vi "PWM_Write.vi"(8 "error in (no error)":errorcluster, 9 "DC":u8(slide) scale=0.0..255.0, 10 "Pin":u8=4 min=4 max=40, 11 "VISA resource name":refnum<visa-resource-name>) -> (0 "error out":errorcluster, 3 "VISA resource name out":refnum<visa-resource-name>)   [LabVIEW 2025]
panel:
  in  "DC%":u8(slide) scale=0.0..100.0
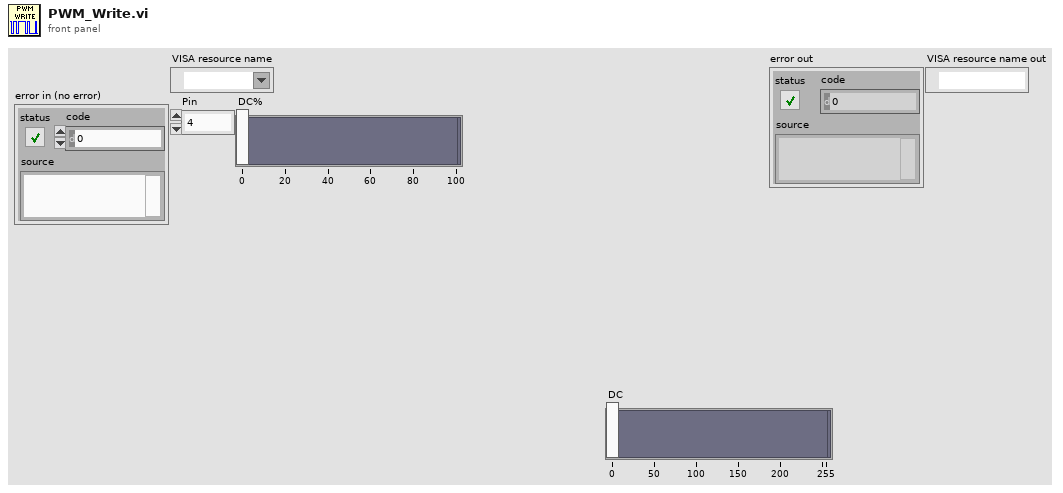
[diagram p1: front panel]
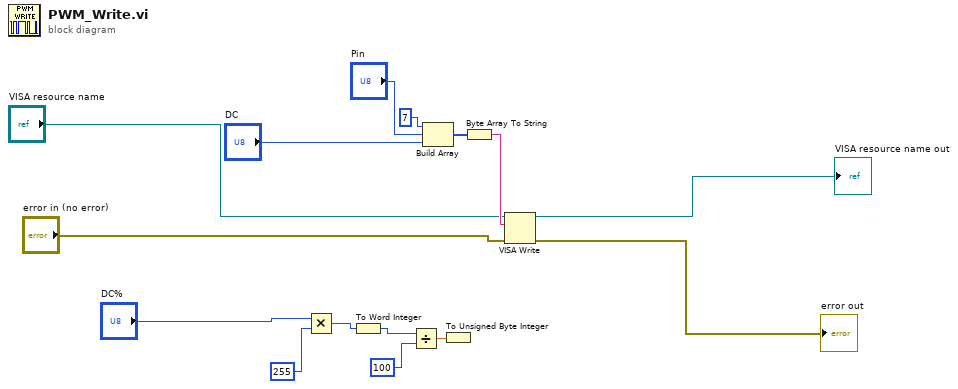
[diagram p0: block diagram]
diagram:
  n1 = Multiply(x="DC%", y=i16 255) -> (x*y=w7:i16)
  n2 = To Word Integer(number=w7) -> (16bit integer=w6:i16)
  n3 = Divide(x=w6, y=u8 100) -> (x/y=w10:dbl)
  n4 = Build Array(u8 7, "Pin", "DC") -> (w13:u8[])
  n5 = To Unsigned Byte Integer(number=w10) -> ()  [unwired: 1 out]
  n6 = Byte Array To String(unsigned byte array=w13) -> (string=w15:string)
  n7 = VISA Write(VISA resource name="VISA resource name", write buffer=w15, error in (no error)="error in (no error)") -> (VISA resource name out=→"VISA resource name out":refnum<visa-resource-name>, error out=→"error out":errorcluster)  [unwired: 1 out]
